vi "ListSUNYFiles.vi"() -> ()   [LabVIEW 2022 SP3]
uses:
  <vilib>/Utility/file.llb/Write Delimited Spreadsheet (string).vi
panel:
  out "Array 2":string[][](array[string])
  in  "Save header":bool
  out "Length":i32
  in  "FIx delete files?":bool
  out "Deletions":path[](array[path])
  in  "Save file":bool
  out "Array":string[][](array[string])
  in  "Folder Path":path=path "\\\\rri-usa.org\\labs/BioMed/Data/SUNY/RawData/LymphNodeData"
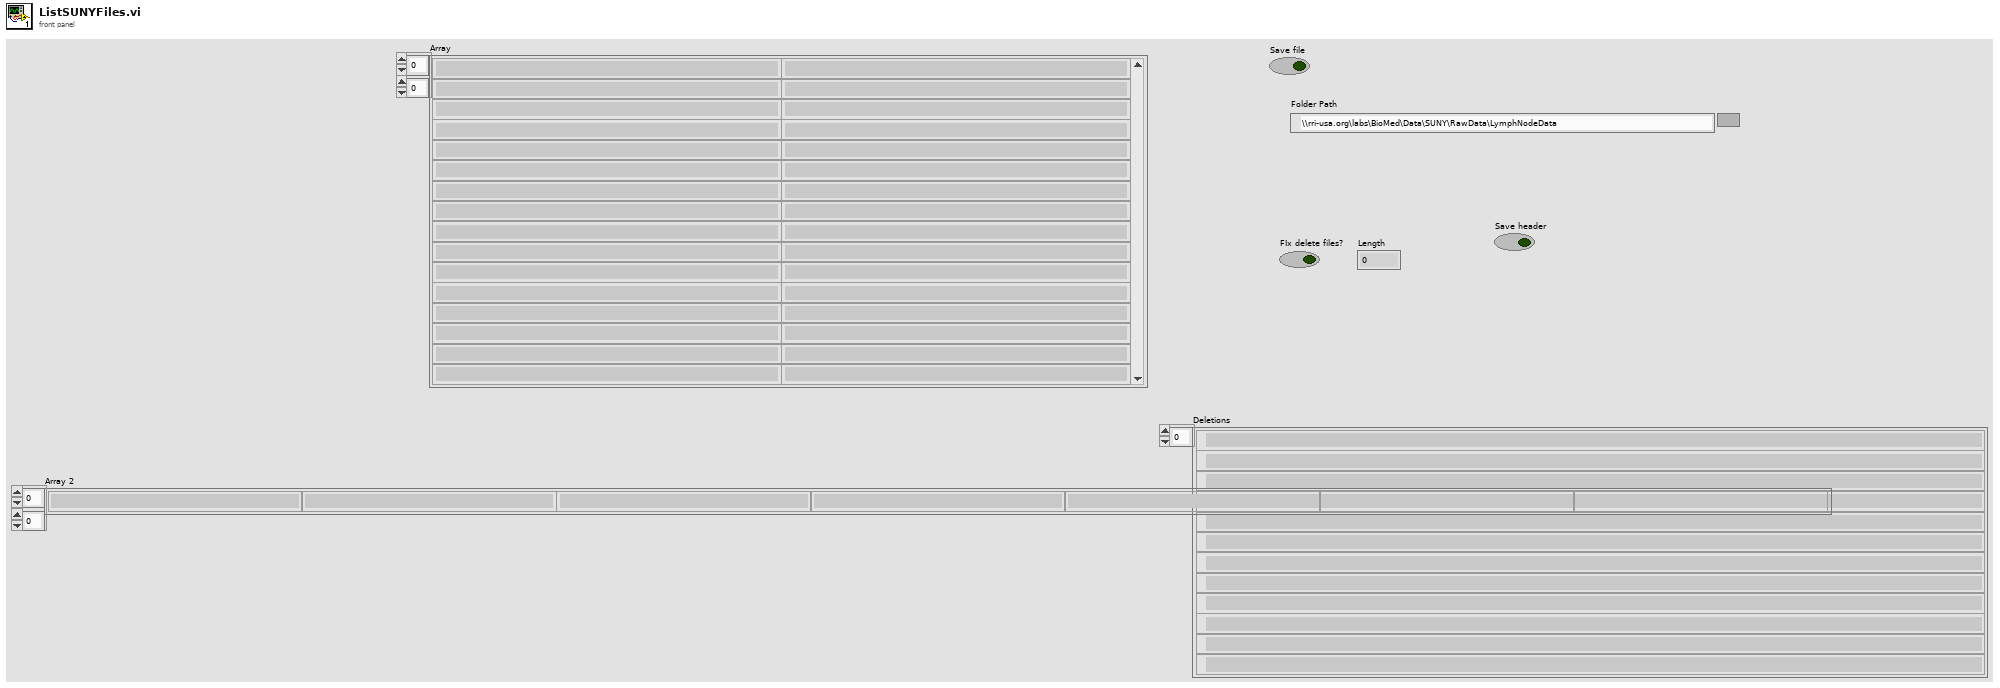
[diagram p1: front panel]
types:
  T1 = typedef "Header.ctl" = cluster{"header info":cluster{"Header":string, "Head length":i16}, "A/D info":cluster{"# rf points per line":u16, "# lines per scan":u16, "sample rate MHz":u16, "# A/D bits":i16, "# bytes per A/D":u16, "TGC Flag":u16, "A/D Type":string}, "Tranducer Info":cluster{"bandwidth":sgl, "center freq":sgl, "start freq":sgl, "ID":i32}, "Scan Info":cluster{"delay":sgl, "pivot distance":sgl, "sector scan angle":sgl, "operator":string, "Scan Mode":string, "location":string}, "Time/Date Info":cluster{"date":string, "time":string}, "RF Info":cluster{"RF file name":string, "RF file att":string, "RF cal file name":string, "RF cal file att":string}, "Patient Info":cluster{"ID":string, "extended ID":string, "age":u16, "sex":string, "previously\nscanned":string, "PSA":sgl, "LOS":u8, "Ethnicty 2":u8, "Race":u8}, "Tissue Type":cluster{"organ":i16, "disease type":i16, "disease location":i16, "IQ_pts":u16, "RcvBuffer":u8, "RcvFrame":u16, "IQBuff":u8, "IQFrame":u16, "IQPage":u8}, "Votage scaling":cluster{"Digitizer (dB)":sgl, "Gain (dB)":sgl, "Atten (dB)":sgl}, "Comment":string, "Misc Info":cluster{"avg num":u16, "c speed":i16, "Div By or SF zones":i16, "XMIT CHS":u8, "RCV CHS":u8, "Xmit angle":sgl}, "Therapy Parameters":cluster{"Theraputic Freq (MHz)":sgl, "Time on (s)":sgl, "Therapy amplitude (mV)":sgl, "Lines Before":u16, "Lines After":u16}, "Scan Settings":cluster{"Energy (uJ or V)":u8, "Damp (Ohm) or Fc":u8, "HP Filt (KHz)":u8, "LP Filt (MHz)":u8, "Gain (db)":u8, "prf (kHz)":sgl, "Distance between\nscan lines (um)":u16, "Distance between\nscan planes (um)":u16, "Scan line gap (um)":sgl, "Scan plane gap (um)":sgl}, "Compression Parameters":cluster{"F1 (MHz)":sgl, "F2 (MHz)":sgl, "% taper":sgl, "duration":sgl}, "Patient Info Xtra":cluster{"First Name":string, "Last Name":string, "Notes":string}, "ROI Box":u16[]}
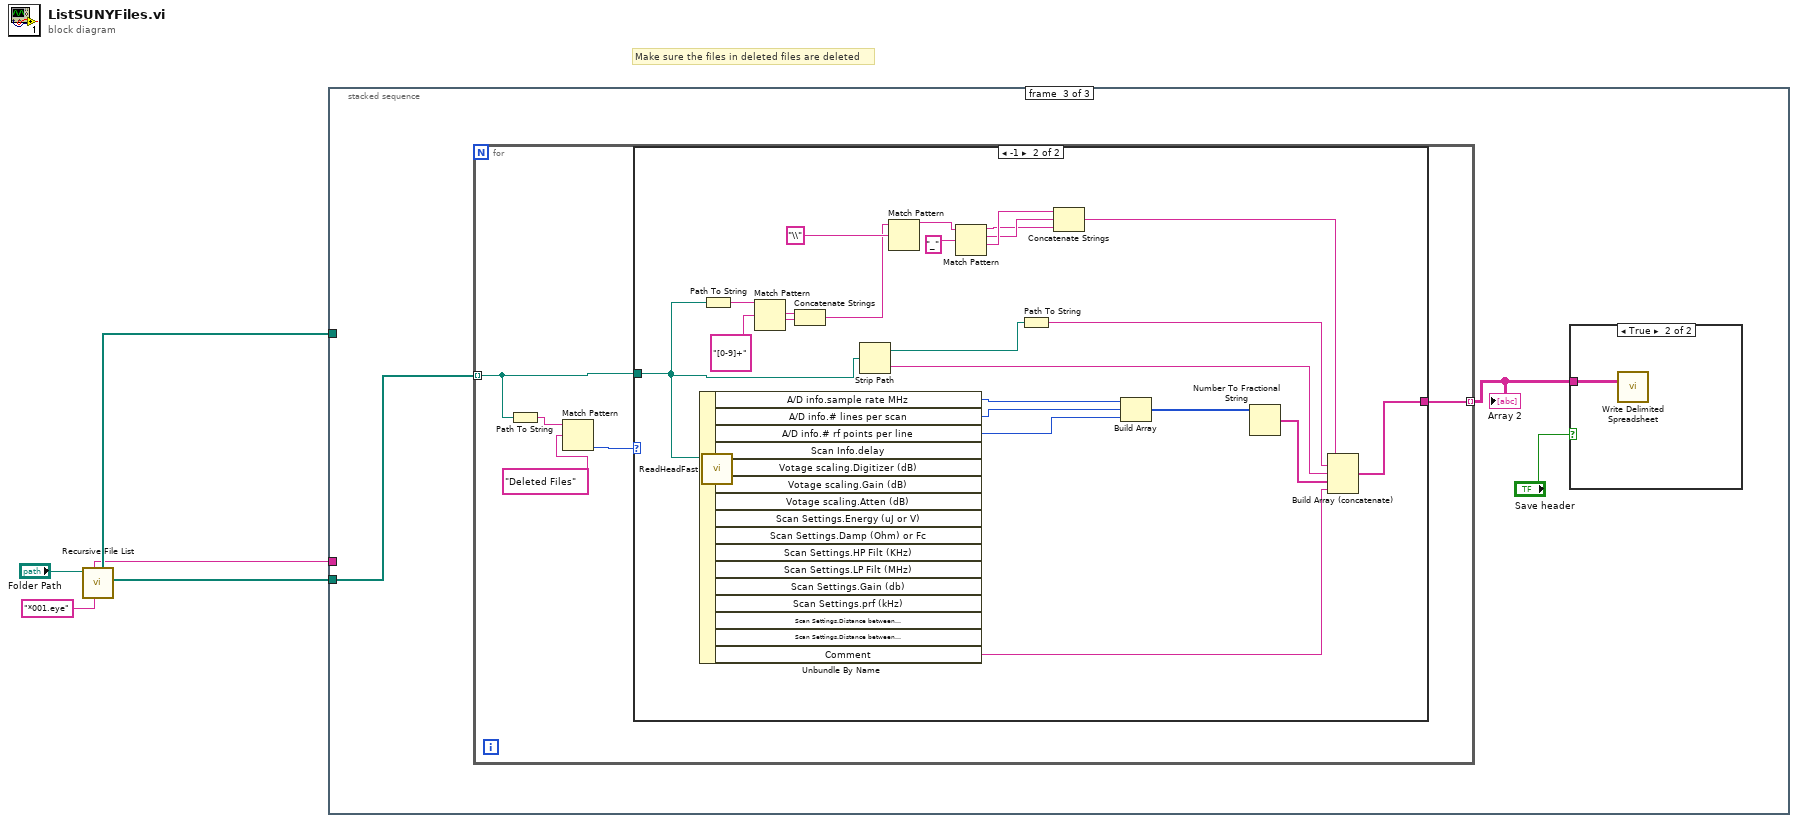
[diagram p0: block diagram]
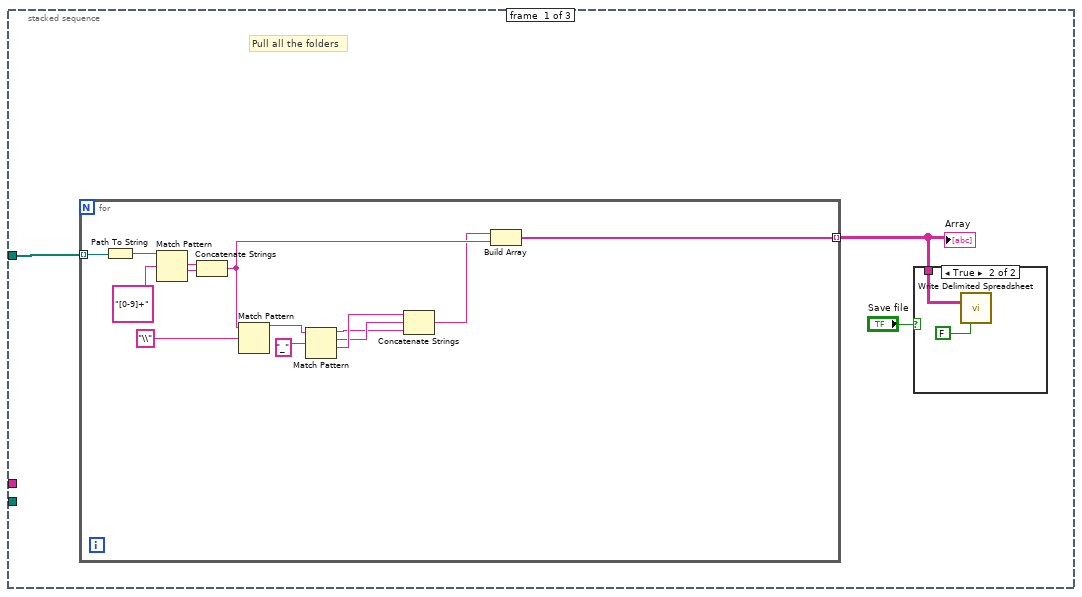
[diagram p2: hidden frame]
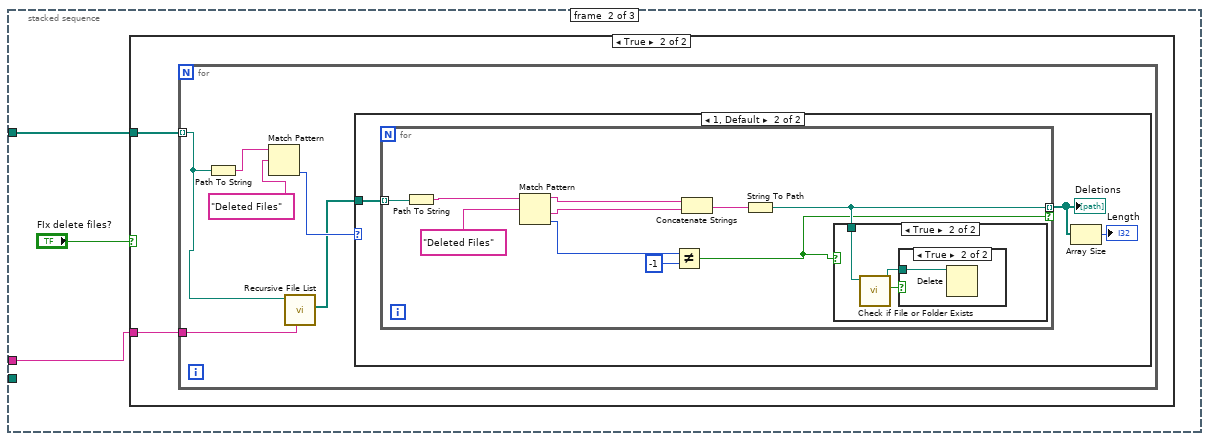
[diagram p4: hidden frame]
diagram:
  w2 = "*001.eye" ("pattern")
  # "Make sure the files in deleted files are deleted"
  n1 = call <vilib>:"Recursive File List.vi"("pattern"=w2, "Folder Path"="Folder Path") -> ("All Files in Dir"=w1:path[], "All Folders"=w3:path[])  [unwired: 5 in, 3 out]
  n2 = stacked-sequence {
    tunnel: w3 -> [w6 w24 _]
    tunnel: w2 -> [_ w25 _]
    tunnel: w1 -> [_ _ w54]
    frame #0 {
      # "Pull all the folders"
      n3 = for {
        tunnel: w6 -> [w23] mode=indexing
        tunnel: [w16] -> w5 mode=indexing
        n4 = Path To String(path=w23) -> (string=w22:string)
        n5 = Match Pattern(string=w22, regular expression="[0-9]+") -> (match substring=w19:string, after substring=w20:string)  [unwired: 1 in, 2 out]
        n6 = Concatenate Strings(w19, w20) -> (w17:string)
        n7 = Match Pattern(string=w17, regular expression="\\") -> (before substring=w15:string)  [unwired: 1 in, 3 out]
        n8 = Match Pattern(string=w15, regular expression="_") -> (before substring=w11:string, match substring=w12:string, after substring=w13:string)  [unwired: 1 in, 1 out]
        n9 = Concatenate Strings(w13, w12, w11) -> (w10:string)
        n10 = Build Array(w10, w17) -> (w16:string[])
      }
      "Array" <- w5
      n11 = case shown="True" "Save file" {
        tunnel: w5 -> [_ w9]
        frame False {
        }
        frame True {
          n12 = call-poly <vilib>:"Write Delimited Spreadsheet.vi"("2D data"=w9, "transpose? (no:F)"=FALSE) -> ()  [unwired: 12 in, 2 out]
        }
      }
    }
    frame #1 {
      n13 = case shown="True" "FIx delete files?" {
        tunnel: w24 -> [_ w28]
        tunnel: w25 -> [_ w27]
        frame False {
        }
        frame True {
          n14 = for {
            tunnel: w28 -> [w31] mode=indexing
            tunnel: w27 -> [w30]
            n15 = Path To String(path=w31) -> (string=w34:string)
            n16 = Match Pattern(string=w34, regular expression="Deleted Files") -> (offset past match=w32:i32)  [unwired: 1 in, 3 out]
            n17 = call <vilib>:"Recursive File List.vi"("pattern"=w30, "Folder Path"=w31) -> ("All Files in Dir"=w29:path[])  [unwired: 5 in, 4 out]
            n18 = case shown="1, Default" w32 {
              tunnel: w29 -> [_ w37]
              frame -1 {
              }
              frame 1, Default {
                n19 = for {
                  tunnel: w37 -> [w47] mode=indexing
                  tunnel: [w39] -> w36 mode=indexing if=w38
                  n20 = Path To String(path=w47) -> (string=w46:string)
                  n21 = Match Pattern(string=w46, regular expression="Deleted Files") -> (before substring=w44:string, after substring=w43:string, offset past match=w41:i32)  [unwired: 1 in, 1 out]
                  n22 = Not Equal?(x=w41, y=-1) -> (x != y?=w38:bool)
                  n23 = Concatenate Strings(w44, w43) -> (w42:string)
                  n24 = String To Path(string=w42) -> (path=w39:path)
                  n25 = case shown="True" w38 {
                    tunnel: w39 -> [_ w49]
                    frame False {
                    }
                    frame True {
                      n26 = call <vilib>:"Check if File or Folder Exists.vi"("path"=w49) -> ("file or folder exists?"=w50:bool, "dup path"=w48:path)  [unwired: 8 in, 1 out]
                      n27 = case shown="True" w50 {
                        tunnel: w48 -> [_ w51]
                        frame False {
                        }
                        frame True {
                          n28 = Delete(path (use dialog)=w51) -> ()  [unwired: 4 in, 3 out]
                        }
                      }
                    }
                  }
                }
                "Deletions" <- w36
                n29 = Array Size(array=w36) -> (size(s)=→"Length":i32)
              }
            }
          }
        }
      }
    }
    frame #2 {
      n30 = for {
        tunnel: w54 -> [w58] mode=indexing
        tunnel: [w56] -> w52 mode=indexing
        n31 = Path To String(path=w58) -> (string=w60:string)
        n32 = Match Pattern(string=w60, regular expression="Deleted Files") -> (offset past match=w57:i32)  [unwired: 1 in, 3 out]
        n33 = case shown="-1" w57 {
          tunnel: w58 -> [_ w72]
          tunnel: [_ w77] -> w56
          frame 0, Default {
          }
          frame -1 {
            n34 = call "ReadHeadFast.vi"("new file path"=w72) -> ("Header In"=w84:T1)  [unwired: 7 in, 3 out]
            n35 = Unbundle By Name(w84) -> ("A/D info.sample rate MHz"=w83:u16, "A/D info.# lines per scan"=w82:u16, "A/D info.# rf points per line"=w81:u16, "Comment"=w78:string)  [unwired: 12 out]
            n36 = Path To String(path=w72) -> (string=w76:string)
            n37 = Match Pattern(string=w76, regular expression="[0-9]+") -> (match substring=w73:string, after substring=w74:string)  [unwired: 1 in, 2 out]
            n38 = Concatenate Strings(w73, w74) -> (w63:string)
            n39 = Strip Path(path=w72) -> (stripped path=w62:path, name=w71:string)
            n40 = Match Pattern(string=w63, regular expression="\\") -> (before substring=w69:string)  [unwired: 1 in, 3 out]
            n41 = Match Pattern(string=w69, regular expression="_") -> (before substring=w65:string, match substring=w66:string, after substring=w67:string)  [unwired: 1 in, 1 out]
            n42 = Path To String(path=w62) -> (string=w61:string)
            n43 = Concatenate Strings(w67, w66, w65) -> (w64:string)
            n44 = Build Array(w83, w82, w81) -> (w80:u16[])
            n45 = Number To Fractional String(number=w80) -> (F-format string=w79:string[])  [unwired: 3 in]
            n46 = Build Array (concatenate)(w64, w61, w71, w79, w78) -> (w77:string[])
          }
        }
      }
      "Array 2" <- w52
      n47 = case shown="True" "Save header" {
        tunnel: w52 -> [_ w55]
        frame False {
        }
        frame True {
          n48 = call-poly <vilib>:"Write Delimited Spreadsheet.vi"("2D data"=w55) -> ()  [unwired: 13 in, 2 out]
        }
      }
    }
  }
